vi "RTcodeRemoveLater.vi"() -> ()   [LabVIEW 2018]
uses:
  <vilib>/FPGAPlugInAG/cRIO-9049/niLvFpga_Open_cRIO-9049.vi
  <vilib>/rvi/interface/common/dynamic/niFpgaDynamicAddResources.vi
  <vilib>/Utility/error.llb/Error Cluster From Error Code.vi
  <vilib>/rvi/errors/niLvFpgaAdjustHostInterfaceError.vi
  <vilib>/FPGAPlugInAG/Dynamic/niLvFpga_Close_Dynamic.vi
  <vilib>/rvi/interface/nirviOpenFPGA/nirviOpenFPGA.xnode
  fpgaInterface/NiFpga_mainFPGA.lvbitx
  <vilib>/rvi/interface/nirviMethod/nirviMethod.xnode
  <vilib>/rvi/interface/nirviReadWriteControl/nirviReadWriteControl.xnode
  <vilib>/rvi/interface/nirviCloseFPGA/nirviCloseFPGA.xnode
  <vilib>/FPGAPlugInAG/Dynamic/niLvFpga_ReadFifo_Dynamic.vi
  <vilib>/rvi/errors/niLvFpgaMergeErrorWithErrorCode.vi
  NiFpgaLv.dll
  <vilib>/rvi/interface/Simulation/niFpgaSimulationCallBeginRW.vi
panel:
  out "Elements Remaining 2":u32
  out "stop":bool
  out "readFifoNow":bool
  out "Data 2":u16[](array[numeric])
  out "Elements Remaining":u32
  in  "error in":errorcluster
  out "error out":errorcluster
  out "Data":u16[](array[numeric])
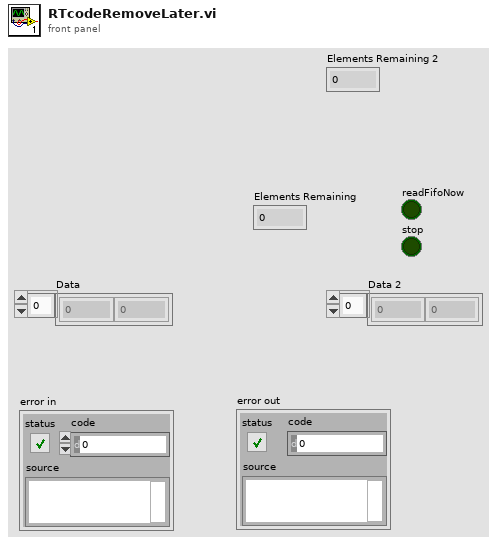
[diagram p1: front panel]
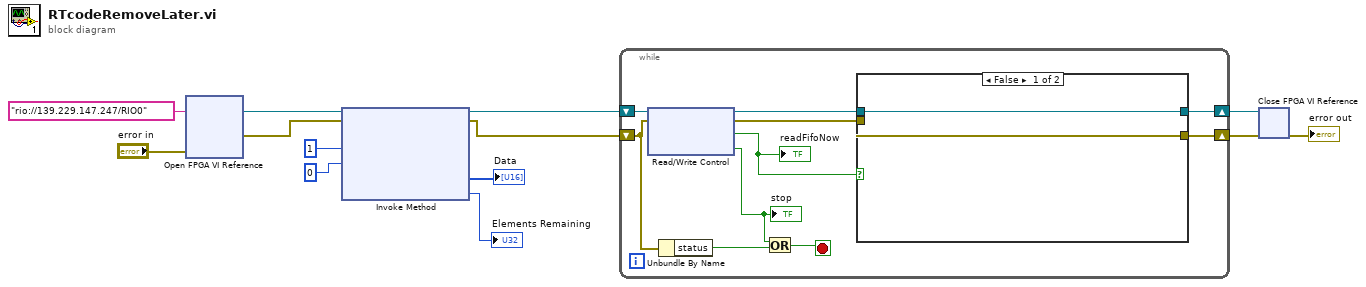
[diagram p0: block diagram]
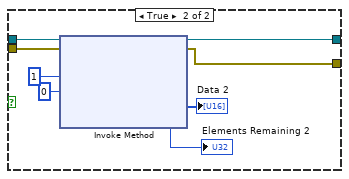
[diagram p2: hidden frame]
diagram:
  n1 = xnode "Open FPGA VI Reference"("error in"="error in", "resource name"=tag "rio://139.229.147.247/RIO0") -> ("FPGA VI Reference Out"=w12:refnum<k20>, "error out"=w11:errorcluster)
  n2 = xnode "Invoke Method"("FPGA VI Reference In"=w12, "error in"=w11, "Number of Elements"=u32 1, "Timeout (ms)"=0) -> ("FPGA VI Reference Out"=w5:refnum<k20>, "error out"=w4:errorcluster, "Data"=→"Data":u16[], "Elements Remaining"=→"Elements Remaining":u32)
  n3 = while {
    shift-right: [w19] -> w2
    shift-left: w5 -> [w23]
    shift-right: [w18] -> w1
    shift-left: w4 -> [w16]
    stop <- w17 stop-if-true
    n4 = xnode "Read/Write Control"("FPGA VI Reference In"=w23, "error in"=w16) -> ("FPGA VI Reference Out"=w22:refnum<k20>, "error out"=w21:errorcluster, "readFifoNow"=w20:bool, "stop"=w14:bool)
    "readFifoNow" <- w20
    "stop" <- w14
    n5 = Unbundle By Name(w16) -> ("status"=w15:bool)
    n6 = Or(x=w14, y=w15) -> (x .or. y?=w17:bool)
    n7 = case shown="False" w20 {
      tunnel: w22 -> [w25 w33]
      tunnel: w21 -> [w24 w32]
      tunnel: [w25 w30] -> w19
      tunnel: [w24 w29] -> w18
      frame False {
      }
      frame True {
        n8 = xnode "Invoke Method"("FPGA VI Reference In"=w33, "error in"=w32, "Number of Elements"=u32 1, "Timeout (ms)"=0) -> ("FPGA VI Reference Out"=w30:refnum<k20>, "error out"=w29:errorcluster, "Data"=→"Data 2":u16[], "Elements Remaining"=→"Elements Remaining 2":u32)
      }
    }
  }
  n9 = xnode "Close FPGA VI Reference"("FPGA VI Reference In"=w2, "error in"=w1) -> ("error out"=→"error out":errorcluster)
